vi "Clear Hardware.vi"(2 "error in (no error)":errorcluster, 3 "Advanced_DMD in":refnum<class "Advanced_DMD.lvclass">) -> (0 "error out":errorcluster, 1 "Advanced_DMD out":refnum<class "Advanced_DMD.lvclass">)   [LabVIEW 2013, in "Advanced_DMD.lvclass"]
doc: "This VI resets any necessary hardware so that the device will be ready for the next run."
uses:
  Advanced_DMD.lvclass
  Device/Device.lvclass
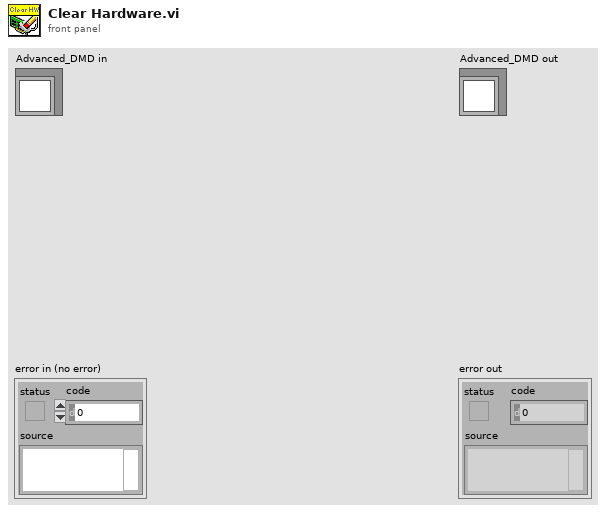
[diagram p1: front panel]
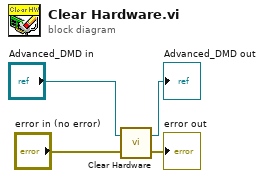
[diagram p0: block diagram]
diagram:
  n1 = call-parent "Clear Hardware.vi"("error in (no error)"="error in (no error)", "Device in"="Advanced_DMD in") -> ("error out"=→"error out":errorcluster, "Device out"=→"Advanced_DMD out":refnum<class "Advanced_DMD.lvclass">)
